vi "Target.vi"   [LabVIEW 2025]
uses:
  <vilib>/eio/utilities/niEioResolveVilibRelativePath.vi
  <vilib>/rvi/interface/RandomDataEmulation/niFpgaRandomDataHandleErrors.vi
  <vilib>/rvi/Memory/Memory_Emulation/nirvimemoryFastEmulation.vi
  <vilib>/rvi/Memory/Memory_Emulation/nirvimemoryEmulation.vi
  <vilib>/rvi/Emulation/niFpgaEmulationIsFPGAContextNoSignature.vi
  <vilib>/rvi/DataTransferAndStorage/Container/Common/niFpgaContainerGetUniqueNameForEmu.vi
  <vilib>/rvi/Emulation/niFpgaProcessEmulError.vi
  <vilib>/rvi/Emulation/niFpgaSctlEmulationGetInTimedLoop.vi
  <vilib>/rvi/errors/nirviReportUnexpectedCaseInternalError (U32).vi
  <vilib>/rvi/DataTransferAndStorage/Container/XNode/niFpgaContainer.xnode
  <vilib>/rvi/interface/RandomDataEmulation/nirviRandomDataFpgaReadWriteTemplate.vi
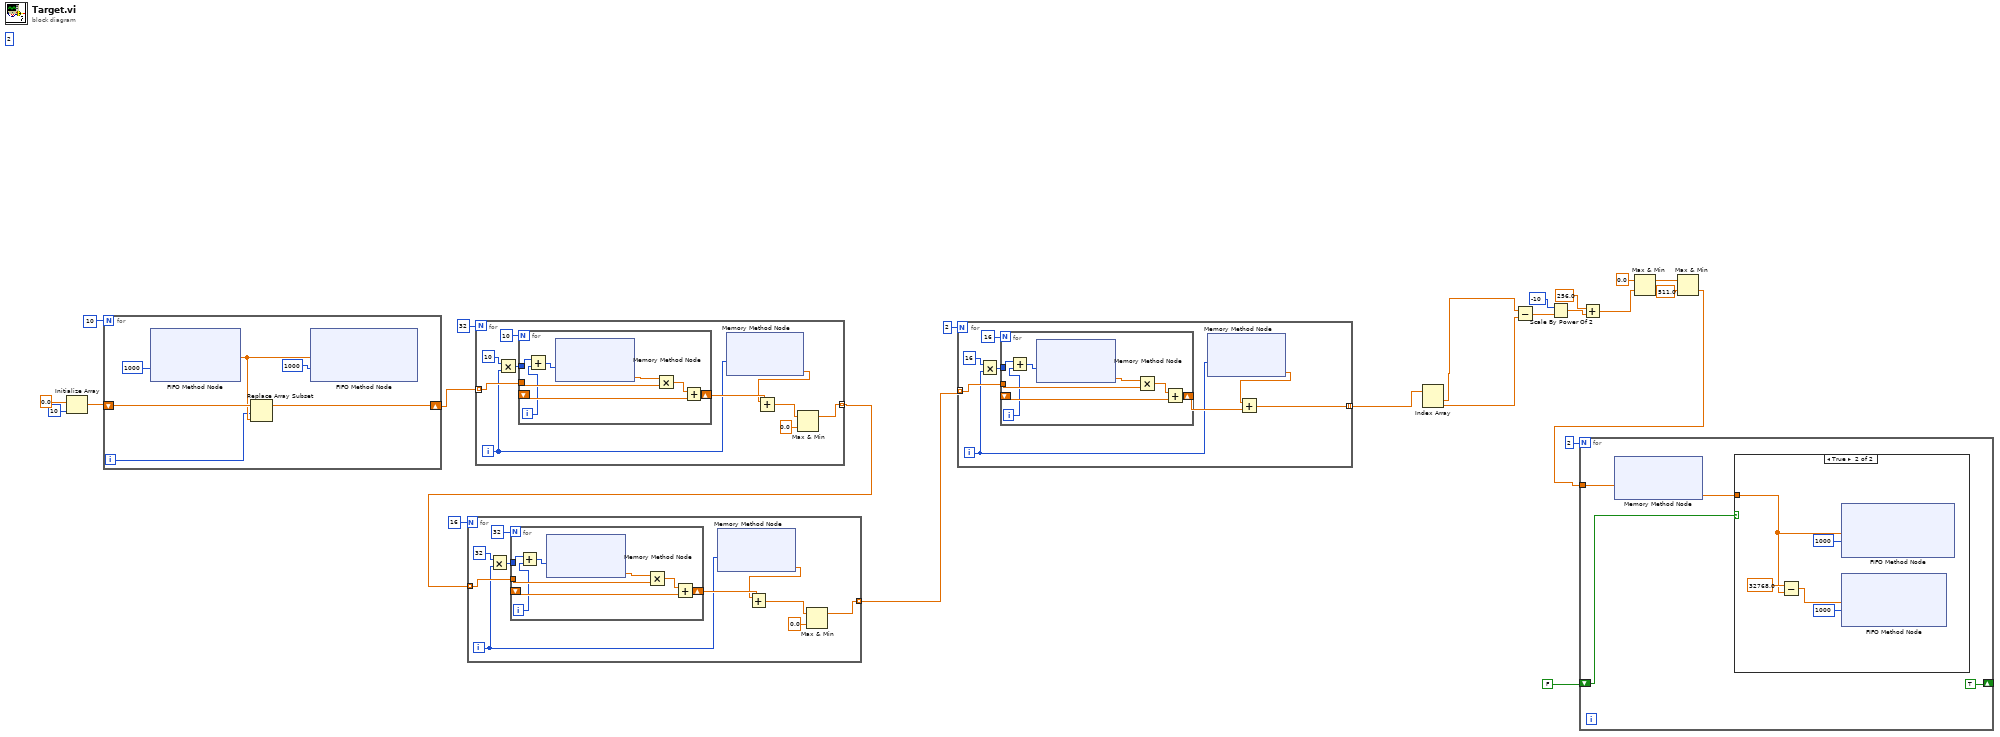
[diagram p0: block diagram]
diagram:
  (unwired) 2
  n1 = Initialize Array(sgl 0.0 ("element"), 10 ("dimension size")) -> (w14:sgl[])
  n2 = for {
    N: 10 -> [_]
    shift-right: [w26] -> w22
    shift-left: w14 -> [w28]
    i -> [w25]
    n3 = xnode ("FIFO Method Node")("Timeout"=1000) -> ("Element"=w27:sgl)  [unwired: 1 in, 2 out]
    n4 = Replace Array Subset(array=w28, new element=w27, index=w25) -> (w26:sgl[])
    n5 = xnode ("FIFO Method Node")("Element"=w27, "Timeout"=1000) -> ()  [unwired: 1 in, 2 out]
  }
  n6 = for {
    N: 32 -> [_]
    tunnel: w22 -> [w40] mode=indexing
    tunnel: [w31] -> w19 mode=indexing
    i -> [w35]
    n7 = Multiply(x=10, y=w35) -> (x*y=w34:i32)
    n8 = for {
      N: 10 -> [_]
      tunnel: w40 -> [w46]
      shift-right: [w45] -> w38
      shift-left: _ -> [w44]
      tunnel: w34 -> [w43]
      i -> [w42]
      n9 = Add(x=w43, y=w42) -> (x+y=w41:i32)
      n10 = xnode ("Memory Method Node")("Address"=w41) -> ("Data"=w48:sgl)  [unwired: 1 in, 1 out]
      n11 = Multiply(x=w48, y=w46) -> (x*y=w47:sgl)
      n12 = Add(x=w47, y=w44) -> (x+y=w45:sgl)
    }
    n13 = xnode ("Memory Method Node")("Address"=w35) -> ("Data"=w37:sgl)  [unwired: 1 in, 1 out]
    n14 = Add(x=w37, y=w38) -> (x+y=w33:sgl)
    n15 = Max & Min(x=w33, y=sgl 0.0) -> (max(x,y)=w31:sgl)  [unwired: 1 out]
  }
  n16 = for {
    N: 16 -> [_]
    tunnel: w19 -> [w58] mode=indexing
    tunnel: [w49] -> w18 mode=indexing
    i -> [w53]
    n17 = Multiply(x=32, y=w53) -> (x*y=w52:i32)
    n18 = for {
      N: 32 -> [_]
      tunnel: w58 -> [w64]
      shift-right: [w63] -> w56
      shift-left: _ -> [w62]
      tunnel: w52 -> [w61]
      i -> [w60]
      n19 = Add(x=w61, y=w60) -> (x+y=w59:i32)
      n20 = xnode ("Memory Method Node")("Address"=w59) -> ("Data"=w66:sgl)  [unwired: 1 in, 1 out]
      n21 = Multiply(x=w66, y=w64) -> (x*y=w65:sgl)
      n22 = Add(x=w65, y=w62) -> (x+y=w63:sgl)
    }
    n23 = xnode ("Memory Method Node")("Address"=w53) -> ("Data"=w55:sgl)  [unwired: 1 in, 1 out]
    n24 = Add(x=w55, y=w56) -> (x+y=w50:sgl)
    n25 = Max & Min(x=w50, y=sgl 0.0) -> (max(x,y)=w49:sgl)  [unwired: 1 out]
  }
  n26 = for {
    N: 2 -> [_]
    tunnel: w18 -> [w74] mode=indexing
    tunnel: [w67] -> w17 mode=indexing
    i -> [w69]
    n27 = Multiply(x=16, y=w69) -> (x*y=w68:i32)
    n28 = for {
      N: 16 -> [_]
      tunnel: w74 -> [w80]
      shift-right: [w79] -> w72
      shift-left: _ -> [w78]
      tunnel: w68 -> [w77]
      i -> [w76]
      n29 = Add(x=w77, y=w76) -> (x+y=w75:i32)
      n30 = xnode ("Memory Method Node")("Address"=w75) -> ("Data"=w82:sgl)  [unwired: 1 in, 1 out]
      n31 = Multiply(x=w82, y=w80) -> (x*y=w81:sgl)
      n32 = Add(x=w81, y=w78) -> (x+y=w79:sgl)
    }
    n33 = xnode ("Memory Method Node")("Address"=w69) -> ("Data"=w71:sgl)  [unwired: 1 in, 1 out]
    n34 = Add(x=w71, y=w72) -> (x+y=w67:sgl)
  }
  n35 = Index Array(array=w17) -> (element #1=w13:sgl, element #2=w12:sgl)  [unwired: 2 in]
  n36 = Subtract(x=w13, y=w12) -> (x-y=w11:sgl)
  n37 = Scale By Power Of 2(n=i16 -10, x=w11) -> (x*2^n=w9:sgl)
  n38 = Add(x=sgl 256.0, y=w9) -> (x+y=w7:sgl)
  n39 = Max & Min(x=sgl 0.0, y=w7) -> (max(x,y)=w5:sgl)  [unwired: 1 out]
  n40 = Max & Min(x=w5, y=sgl 511.0) -> (min(x,y)=w2:sgl)  [unwired: 1 out]
  n41 = for {
    N: 2 -> [_]
    tunnel: w2 -> [w86]
    shift-right: [TRUE] -> _
    shift-left: FALSE -> [w85]
    n42 = xnode ("Memory Method Node")("Address"=w86) -> ("Data"=w83:sgl)  [unwired: 1 in, 1 out]
    n43 = case shown="True" w85 {
      tunnel: w83 -> [_ w87]
      frame False {
      }
      frame True {
        n44 = Subtract(x=sgl 32768.0, y=w87) -> (x-y=w91:sgl)
        n45 = xnode ("FIFO Method Node")("Element"=w87, "Timeout"=1000) -> ()  [unwired: 1 in, 2 out]
        n46 = xnode ("FIFO Method Node")("Element"=w91, "Timeout"=1000) -> ()  [unwired: 1 in, 2 out]
      }
    }
  }
